vi "Cmd_SetPosition.vi"(11 "Msg Data":variant) -> ()   [LabVIEW 2011]
uses:
  Main/Motors/MotorCmd_SetPosition.ctl
  Main/Motors/MotorAxisEnum.ctl
  PIAxisInfoGlobal.vi
  Main/GlobalVariables.vi
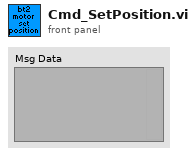
[diagram p1: front panel]
types:
  T1 = typedef "MotorCmd_SetPosition.ctl" = cluster{"Position":dbl, "Speed":sgl, "Instant?":bool, "Motor Axis":T2}
  T2 = typedef "MotorAxisEnum.ctl" = enum16{"no axis", "magrot", "magpos", "px", "py", "pz", "camx", "camy"}
  T3 = typedef "MotorConfigType.ctl" = cluster{"Offset":T4, "Maximum pos":T4, "Min limited?":T6, "Max limited?":T6, "Has velocity support":T6, "Default velocity":T4}
  T4 = typedef "MotorPosType.ctl" = cluster{"Magnet Z":dbl, "Magnet rotation":dbl, "Camera":T5, "Piezo XY":T5, "Piezo Z":dbl, "Coil XY":T5}
  T5 = typedef "XYf.ctl" = cluster{"X":sgl, "Y":sgl}
  T6 = typedef "MotorPosFlagsType.ctl" = cluster{"Magnet Z":bool, "Magnet rotation":bool, "Camera":cluster{"X":bool, "Y":bool}, "Piezo XY":cluster{"X":bool, "Y":bool}, "Piezo Z":bool, "Coil XY":cluster{"X":bool, "Y":bool}}
  T7 = cluster{"Magnet Z":i16, "Magnet rotation":i16, "Camera":cluster{"X":i16, "Y":i16}, "Piezo XY":cluster{"X":i16, "Y":i16}, "Piezo Z":i16, "Coil XY":cluster{"X":i16, "Y":i16}}
  T8 = typedef "PI_Axis.ctl" = cluster{"System #":i32, "Axis ID":string, "Multiplier":dbl}
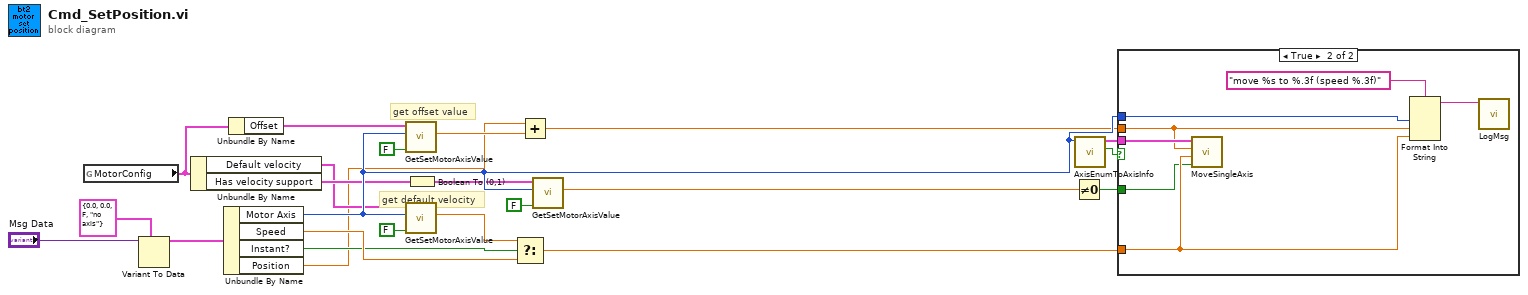
[diagram p0: block diagram]
diagram:
  # "get offset value"
  # "get default velocity"
  n1 = global read "GlobalVariables.vi" "MotorConfig"() -> (w23:T3)
  n2 = Variant To Data(type=T1 {"Position"=0.0, "Speed"=0.0, "Instant?"=FALSE, "Motor Axis"=enum."no axis"} ("SetMotorPosCmdData"), Variant="Msg Data") -> (data=w2:T1)  [unwired: 1 in, 1 out]
  n3 = Unbundle By Name(w23) -> ("Default velocity"=w11:T4, "Has velocity support"=w13:T6)
  n4 = Unbundle By Name(w2) -> ("Motor Axis"=w15:T2, "Speed"=w18:sgl, "Instant?"=w17:bool, "Position"=w4:dbl)
  n5 = Unbundle By Name(w23) -> ("Offset"=w5:T4)
  n6 = call "GetSetMotorAxisValue.vi"("set? (T)"=FALSE, "axis"=w15, "Motorpos in"=w5) -> ("pos (out)"=w7:dbl)  [unwired: 7 in, 1 out]
  n7 = call "GetSetMotorAxisValue.vi"("set? (T)"=FALSE, "axis"=w15, "Motorpos in"=w11) -> ("pos (out)"=w19:dbl)  [unwired: 7 in, 1 out]
  n8 = Boolean To (0,1)(Boolean=w13) -> (0, 1=w14:T7)
  n9 = Select(t=w19, s=w17, f=w18) -> (s? t:f=w20:dbl)
  n10 = Add(x=w4, y=w7) -> (x+y=w9:dbl)
  n11 = call "GetSetMotorAxisValue.vi"("set? (T)"=FALSE, "axis"=w15, "Motorpos in"=w14) -> ("pos (out)"=w21:dbl)  [unwired: 7 in, 1 out]
  n12 = Not Equal To 0?(x=w21) -> (x != 0?=w22:bool)
  n13 = call "AxisEnumToAxisInfo.vi"("Motor Axis"=w15) -> ("Valid axis?"=w8:bool, "Axis info"=w10:T8)  [unwired: 6 in, 3 out]
  n14 = case shown="True" w8 {
    tunnel: w9 -> [_ w24]
    tunnel: w10 -> [_ w27]
    tunnel: w15 -> [_ w29]
    tunnel: w20 -> [_ w26]
    tunnel: w22 -> [_ w25]
    frame False {
    }
    frame True {
      n15 = call "MoveSingleAxis.vi"("Set velocity?"=w25, "Velocity"=w26, "Position"=w24, "Axis info"=w27) -> ()  [unwired: 8 in]
      n16 = Format Into String(format string="move %s to %.3f (speed %.3f)", w29, w24, w26) -> (resulting string=w28:string)  [unwired: 2 in, 1 out]
      n17 = call "LogMsg.vi"("msg"=w28) -> ()  [unwired: 11 in]
    }
  }
